vi "PID Reef Align.vi"(6 "Tag ID":dbl=17.0, 7 "Y movement":dbl, 8 "Int per ft":dbl=0.75, 9 "setpoint":dbl=-0.49) -> (0 "PID Happy?":bool, 2 "Robot Velocities Out":cluster{"output":dbl, "y":dbl, "y":dbl}={"output"=0.3376314931743365, "y"=0.0, "y"=0.0})   [LabVIEW 2023]
uses:
  <vilib>/Rock Robotics/WPI/DriverStation/WPI_DriverStationRobotMode2.ctl
  <vilib>/Rock Robotics/Network Tables/NT Read Numeric Array.vi
  <vilib>/Rock Robotics/Network Tables/NT Read Number.vi
  Framework/Robot Global Data.vi
  <vilib>/ptbypt/NI_PtbyPt.lvlib
panel:
  in  "Forward speed":dbl=1.1
  in  "PID Threshold":dbl=5.0
  in  "Deadband Auto":dbl=0.075
  in  "Deadband Tele":dbl=0.075
  out "Waveform Chart":cluster{"setpoint":dbl, "output":dbl}(graph)={"setpoint"=-0.5923125736891929, "output"=-0.49}
  in  "PID gains":T1={"proportional gain (Kp)"=3.3, "integral time (Ki)"=0.0, "derivative time (Kd)"=0.19999999999999998} {"derivative time (Kd)" format="%.3f"; "integral time (Ki)" format="%.3f"; "proportional gain (Kp)" format="%.3f"}
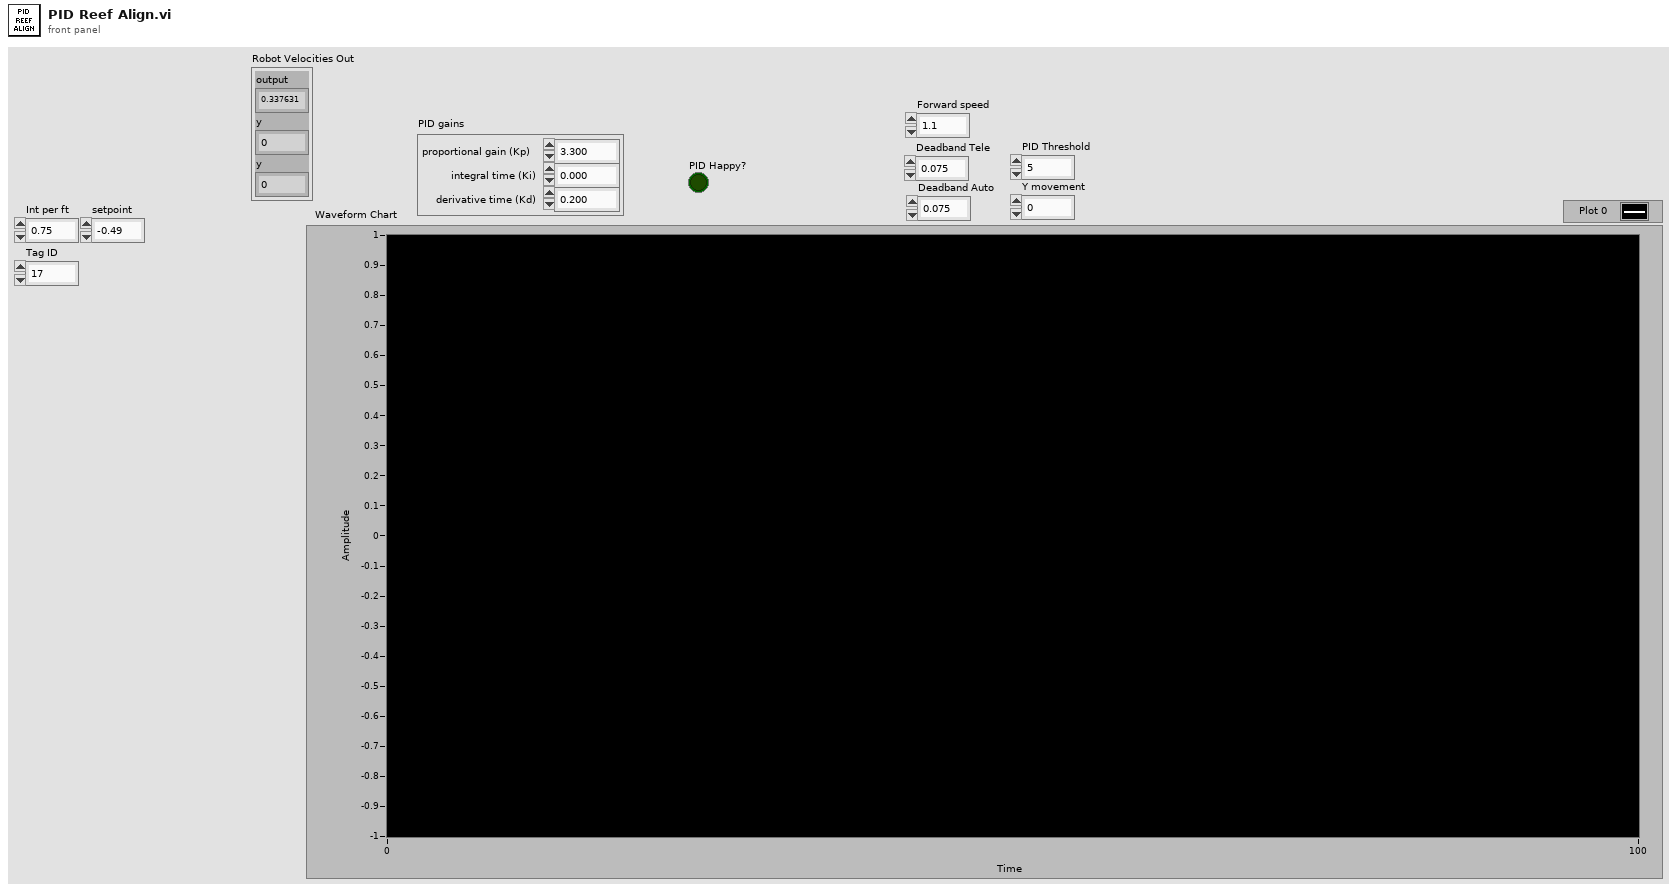
[diagram p1: front panel]
types:
  T1 = cluster{"proportional gain (Kp)":dbl, "integral time (Ki)":dbl, "derivative time (Kd)":dbl}
  T2 = typedef "WPI_DriverStationRobotMode2.ctl" = enum16{"Autonomous Disabled", "Autonomous Enabled", "Teleop Disabled", "Teleop Enabled", "Disconnected", "Finish", "Test Disabled", "Test Enabled", "Emergency Stopped"}
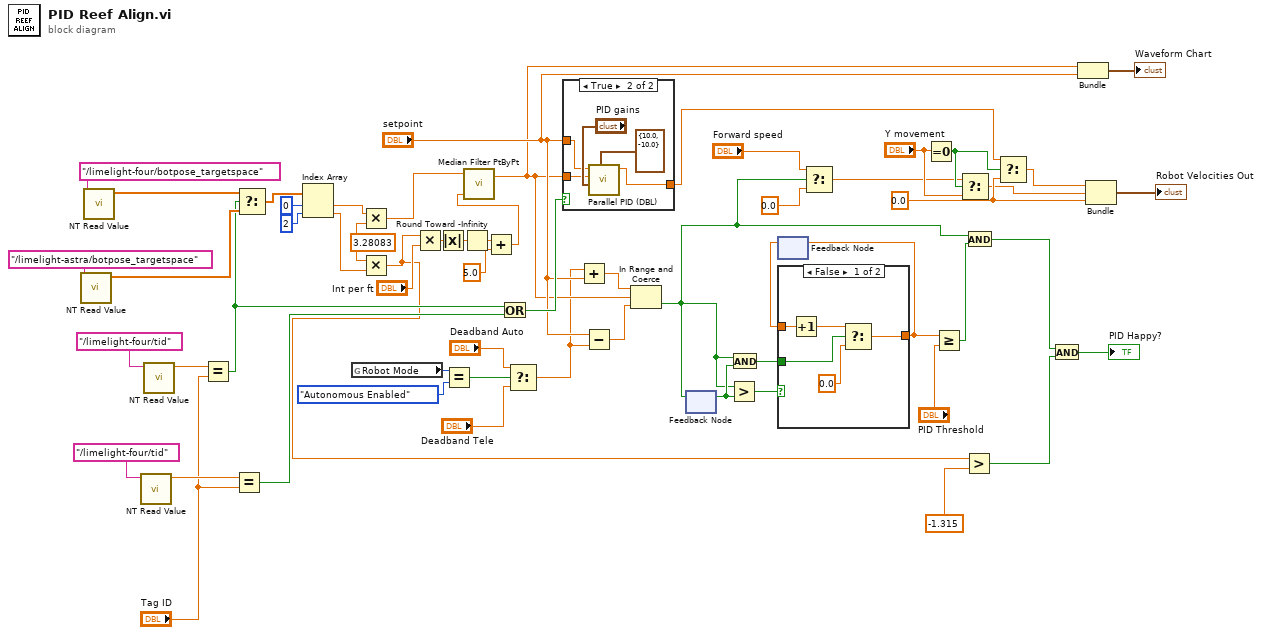
[diagram p0: block diagram]
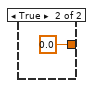
[diagram p2: hidden frame]
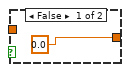
[diagram p3: hidden frame]
diagram:
  w14 = 0.0 ("y")
  w52 = 3.28083 ("x")
  n1 = call-poly <vilib>:"NT Read Value.vi"("name"="/limelight-astra/botpose_targetspace") -> ("value"=w43:dbl[])  [unwired: 8 in, 2 out]
  n2 = call-poly <vilib>:"NT Read Value.vi"("name"="/limelight-four/botpose_targetspace") -> ("value"=w44:dbl[])  [unwired: 8 in, 2 out]
  n3 = call-poly <vilib>:"NT Read Value.vi"("name"="/limelight-four/tid") -> ("value"=w40:dbl)  [unwired: 8 in, 2 out]
  n4 = call-poly <vilib>:"NT Read Value.vi"("name"="/limelight-four/tid") -> ("value"=w55:dbl)  [unwired: 8 in, 2 out]
  n5 = Equal?(x=w55, y="Tag ID") -> (x = y?=w37:bool)
  n6 = Equal?(x=w40, y="Tag ID") -> (x = y?=w38:bool)
  n7 = Select(t=w44, s=w37, f=w43) -> (s? t:f=w42:dbl[])
  n8 = Index Array(array=w42, index #1=0 ("index"), index #2=2 ("index")) -> (element #1=w57:dbl, element #2=w53:dbl)
  n9 = global read "Robot Global Data.vi" "Robot Mode"() -> (w27:T2)
  n10 = Multiply(x=w57, y=w52) -> (x*y=w35:dbl)
  n11 = Multiply(x=w52, y=w53) -> (x*y=w6:dbl)
  n12 = Multiply(x=w6, y="Int per ft") -> (x*y=w50:dbl)
  n13 = Absolute Value(x=w50) -> (abs(x)=w49:dbl)
  n14 = Equal?(x=w27, y=WPI_DriverStationRobotMode2."Autonomous Enabled") -> (x = y?=w25:bool)
  n15 = Round Toward -Infinity(1:w49) -> (0:w48:dbl)
  n16 = Add(x=w48, y=5.0) -> (x+y=w46:dbl)
  n17 = call <vilib>:"Median Filter PtByPt.vi"("rank"=w46, "x"=w35) -> ("Filtered x"=w29:dbl)  [unwired: 2 in, 1 out]
  n18 = Or(x=w37, y=w38) -> (x .or. y?=w36:bool)
  n19 = Select(t="Deadband Auto", s=w25, f="Deadband Tele") -> (s? t:f=w28:dbl)
  n20 = case shown="True" w36 {
    tunnel: w29 -> [_ w63]
    tunnel: "setpoint" -> [_ w62]
    tunnel: [0.0 ("output") w61] -> w15
    frame False {
    }
    frame True {
      n21 = call <vilib>:"Parallel PID (DBL).vi"("output range"=cluster{"high":dbl, "low":dbl} {"high"=10.0, "low"=-10.0}, "PID gains"="PID gains", "process variable"=w63, "setpoint"=w62) -> ("output"=w61:dbl)  [unwired: 4 in, 3 out]
    }
  }
  n22 = Add(x=w28, y="setpoint") -> (x+y=w32:dbl)
  n23 = Subtract(x="setpoint", y=w28) -> (x-y=w30:dbl)
  n24 = In Range and Coerce(upper limit=w32, x=w29, lower limit=w30) -> (In Range?=w8:bool)  [unwired: 1 out]
  n25 = feedback #1() -> (w22:bool)  [unwired: 1 in]
  n26 = feedback-in #1(w8) -> ()
  n27 = Greater?(x=w8, y=w22) -> (0:w21:bool)
  n28 = And(x=w8, y=w22) -> (x .and. y?=w19:bool)
  n29 = feedback #2() -> (w20:dbl)  [unwired: 1 in]
  n30 = case shown="False" w21 {
    tunnel: [w69 0.0] -> w18
    tunnel: w20 -> [w70 _]
    tunnel: w19 -> [w67 _]
    frame False {
      n31 = Increment(x=w70) -> (x+1=w66:dbl)
      n32 = Select(t=w66, s=w67, f=0.0) -> (s? t:f=w69:dbl)
    }
    frame True {
    }
  }
  n33 = feedback-in #2(w18) -> ()
  n34 = Select(t="Forward speed", s=w8, f=0.0) -> (s? t:f=w9:dbl)
  n35 = Equal To 0?(x="Y movement") -> (x = 0?=w10:bool)
  n36 = Greater Or Equal?(x=w18, y="PID Threshold") -> (x >= y?=w16:bool)
  n37 = Select(t=w9, s=w10, f="Y movement") -> (s? t:f=w12:dbl)
  n38 = Greater?(x=w6, y=-1.315) -> (0:w3:bool)
  n39 = And(x=w8, y=w16) -> (x .and. y?=w4:bool)
  n40 = Select(t=w15, s=w10, f=w14) -> (s? t:f=w13:dbl)
  n41 = And(x=w4, y=w3) -> (x .and. y?=→"PID Happy?":bool)
  n42 = Bundle("Filtered x"=w29, "setpoint"="setpoint") -> (→"Waveform Chart":cluster{"Filtered x":dbl, "setpoint":dbl})  [unwired: 1 in]
  n43 = Bundle("y"=w13, "Y movement"=w12, "y"=w14) -> (→"Robot Velocities Out":cluster{"y":dbl, "Y movement":dbl, "y":dbl})  [unwired: 1 in]
